vi "Word_Insert_New_Line.vi"(0 "Word._Document":refnum<k7>, 1 "font":T1 {"font size" format="%.2f"; "strike through" items=["Unchanged", "Yes", "No"]; "underline" items=["Unchanged", "Yes", "No"]; "italic" items=["Unchanged", "Yes", "No"]; "bold" items=["Unchanged", "Yes", "No"]}, 2 "Style":string, 5 "Text":string, 7 "Start":i32, 9 "End":i32, 11 "Error in (no error)":errorcluster, 12 "Insertion point":u16(ring)=1 items=["begining of document", "end of document", "bookmark", "custom"], 13 "Bookmark name":string) -> (4 "ActiveDocument out":refnum<k7>, 8 "Start out":i32, 10 "End out":i32, 15 "Error out":errorcluster={"status"=FALSE, "code"=0, "source"=" "})   [LabVIEW 2010, in "NI_ReportGenerationToolkit.lvlib"]
uses:
  <vilib>/addons/_office/NI_ReportGenerationToolkit.lvlib
  <vilib>/addons/_office/_exclsub.llb/font.ctl
panel:
  # "Content"
  # "Position"
  # "Output"
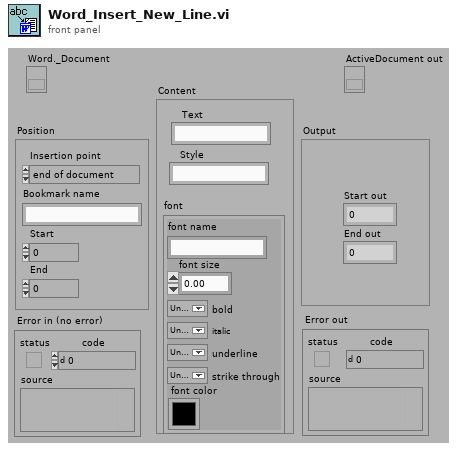
[diagram p1: front panel]
types:
  T1 = typedef "NI_ReportGenerationToolkit.lvlib/font.ctl" = cluster{"font name":string, "font size":dbl, "bold":u16, "italic":u16, "underline":u16, "strike through":u16, "font color":u32}
  T2 = cluster{"Alignment":enum16{"Left", "Centered", "Right", "Justify"}, "Left":dbl, "Right":dbl, "Special":enum16{"(none)", "First line", "Hanging"}, "By":dbl, "Before":dbl, "After":dbl, "Line spacing":enum16{"Single", "1,5 lines", "Double", "At least", "Exactly", "Multiple"}, "At":dbl}
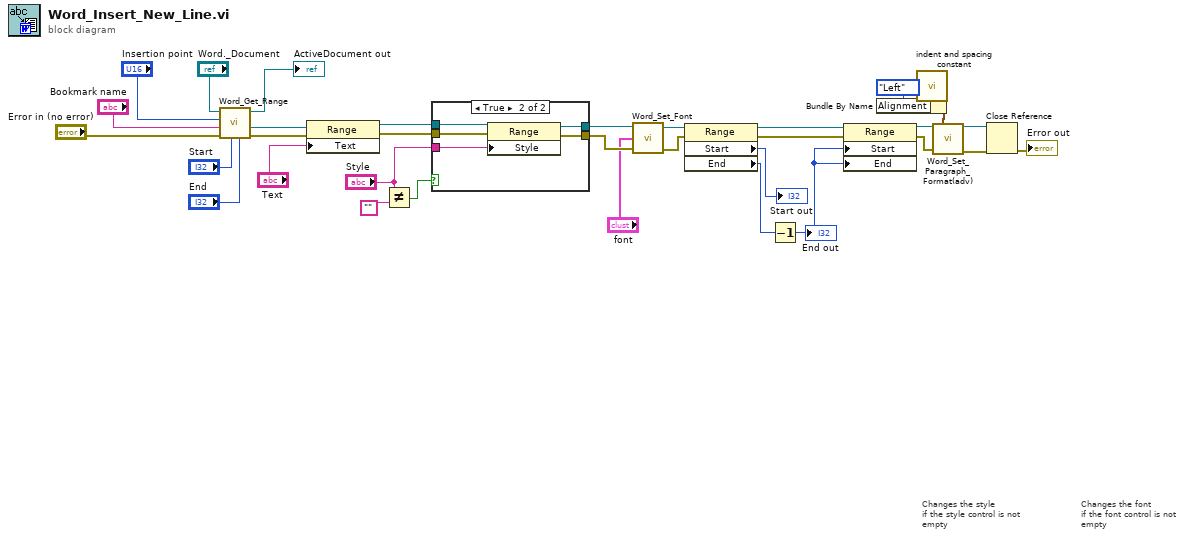
[diagram p0: block diagram]
diagram:
  # "Changes the font\nif the font control is not\nempty"
  # "Changes the style\nif the style control is not\nempty"
  n1 = call <vilib>:"Word_Get_Range.vi"("end"="End", "start"="Start", "error in"="Error in (no error)", "bookmark name"="Bookmark name", "insertion point"="Insertion point", "document in"="Word._Document") -> ("error out (no error)"=w27:errorcluster, "range"=w26:refnum<k7>, "document out"=→"ActiveDocument out":refnum<k7>)  [unwired: 3 out]
  n2 = property class="Range"(reference=w26, error in=w27, "Text"="Text") -> (reference out=w19:refnum<k7>, error out=w18:errorcluster)
  n3 = Not Equal?(x="Style", y="") -> (x != y?=w14:bool)
  n4 = case shown="True" w14 {
    tunnel: w19 -> [w35 w40]
    tunnel: w18 -> [w34 w39]
    tunnel: [w35 w38] -> w17
    tunnel: [w34 w37] -> w16
    tunnel: "Style" -> [_ w36]
    frame False {
    }
    frame True {
      n5 = property class="Range"(reference=w40, error in=w39, "Style"=w36) -> (reference out=w38:refnum<k7>, error out=w37:errorcluster)
    }
  }
  n6 = call <vilib>:"Word_Set_Font.vi"("Range in"=w17, "font"="font", "Error in"=w16) -> ("Range out"=w25:refnum<k7>, "Error out"=w24:errorcluster)  [unwired: 5 out]
  n7 = property class="Range"(reference=w25, error in=w24) -> (reference out=w10:refnum<k7>, error out=w9:errorcluster, "Start"=→"Start out":i32, "End"=w22:i32)
  n8 = Decrement(x=w22) -> (x-1=w8:i32)
  "End out" <- w8
  n9 = property class="Range"(reference=w10, error in=w9, "Start"=w8, "End"=w8) -> (reference out=w7:refnum<k7>, error out=w6:errorcluster)
  n10 = call <vilib>:"indent and spacing constant.vi"() -> ("indent and spacing"=w3:T2)
  n11 = Bundle By Name(cluster=w3, "Alignment"=enum16{"Left", "Centered", "Right", "Justify"}."Left") -> (w1:T2)
  n12 = call <vilib>:"Word_Set_Paragraph_Format(adv).vi"("Range in"=w7, "Indent and spacing"=w1, "Error in"=w6) -> ("Range out"=w4:refnum<k7>, "Error out"=w5:errorcluster)  [unwired: 2 in, 9 out]
  n13 = Close Reference(reference=w4, error in (no error)=w5) -> (error out=→"Error out":errorcluster)
